vi "Inputs.vi"(8 "error in (no error)":errorcluster, 11 "State in":T1={"State"=enum."Idle", "Start Time"=timestamp(0 s since 1904-01-01), "Configuration"={"Cycle Period"=0.0, "Mettler"={"VISA resource name"="", "Simulated?"=FALSE}, "Scale Type"=""}, "Current Time"=timestamp(0 s since 1904-01-01), "First Iteration"=FALSE, "Data"={"Scale Read(g)"=0.0}, "Process Name"="", "Log Started"=FALSE}) -> (0 "error out":errorcluster, 3 "State out":T1={"State"=enum."Idle", "Start Time"=timestamp(0 s since 1904-01-01), "Configuration"={"Cycle Period"=0.0, "Mettler"={"VISA resource name"="", "Simulated?"=FALSE}, "Scale Type"=""}, "Current Time"=timestamp(0 s since 1904-01-01), "First Iteration"=FALSE, "Data"={"Scale Read(g)"=0.0}, "Process Name"="", "Log Started"=FALSE})   [LabVIEW 2018, in "Sonicator Module.lvlib" / "Sonicator Module Engine.lvlib"]
uses:
  Sonicator Module Engine.lvlib
  State Cluster.ctl
  State Enum.ctl
  Feed Module/Controls/Sonicator Module Settings Cluster.ctl
  Mettler Toledo/Controls/Settings Cluster.ctl
  Tag VIs/Tag FGV Operation Enum.ctl
  Mettler Toledo/Mettler Toledo.lvlib
  Shared Variables/Dynamic Shared Variables.lvlib
  Sonicator Module.lvlib
panel:
  # "Scale Settings"
  # "Scale Settings"
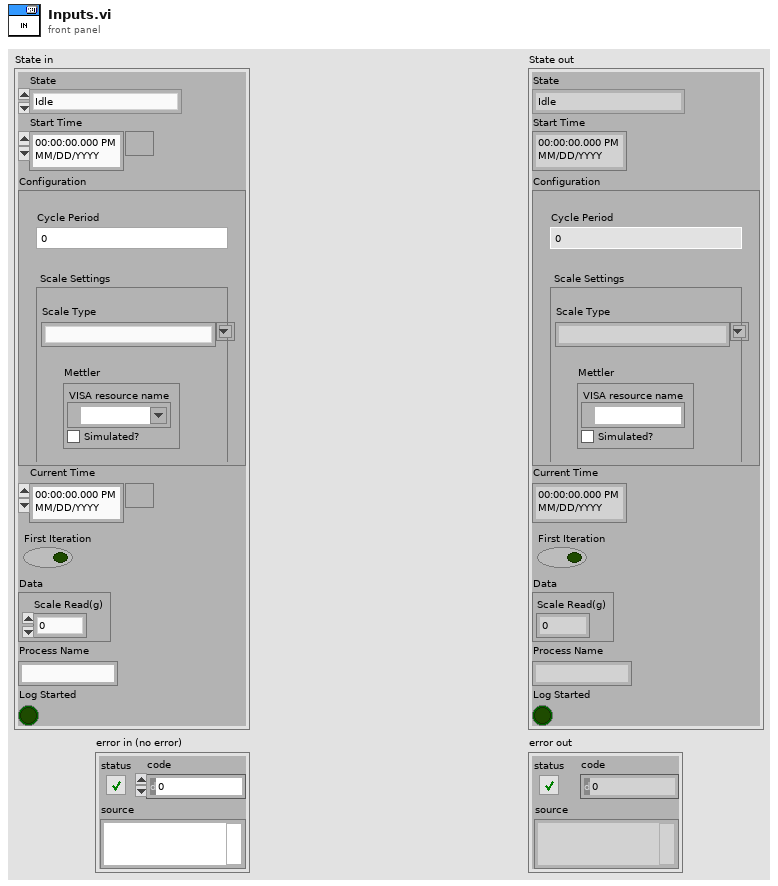
[diagram p1: front panel]
types:
  T1 = typedef "Sonicator Module.lvlib/Sonicator Module Engine.lvlib/State Cluster.ctl" = cluster{"State":T2, "Start Time":timestamp, "Configuration":T3, "Current Time":timestamp, "First Iteration":bool, "Data":cluster{"Scale Read(g)":dbl}, "Process Name":string, "Log Started":bool}
  T2 = typedef "Sonicator Module.lvlib/Sonicator Module Engine.lvlib/State Enum.ctl" = enum16{"Measuring", "Idle"}
  T3 = typedef "Sonicator Module.lvlib/Sonicator Module Settings Cluster.ctl" = cluster{"Cycle Period":dbl, "Mettler":T4, "Scale Type":string}
  T4 = typedef "Mettler Toledo.lvlib/Settings Cluster.ctl" = cluster{"VISA resource name":refnum<visa-resource-name>, "Simulated?":bool}
  T5 = typedef "Tag FGV Operation Enum.ctl" = enum16{"Init", "Set Notification Queue", "Create Tag", "Commit", "Write Tag (Numeric)", "Write Tag (Boolean)", "Read All Tags", "Read One Tag", "Delete Tag Category", "Set Alarm Parameters (Numeric)", "Set Alarm Parameters (Boolean)", "Enable All Alarms", "Disable All Alarms", "Delete All Tags", "Read Alarms", "Ack Alarm", "Read Alarm Parameters (Numeric)", "Read Alarm Parameters (Boolean)"}
  T6 = cluster{"Scale Tag":string, "Output Device Tag":string}
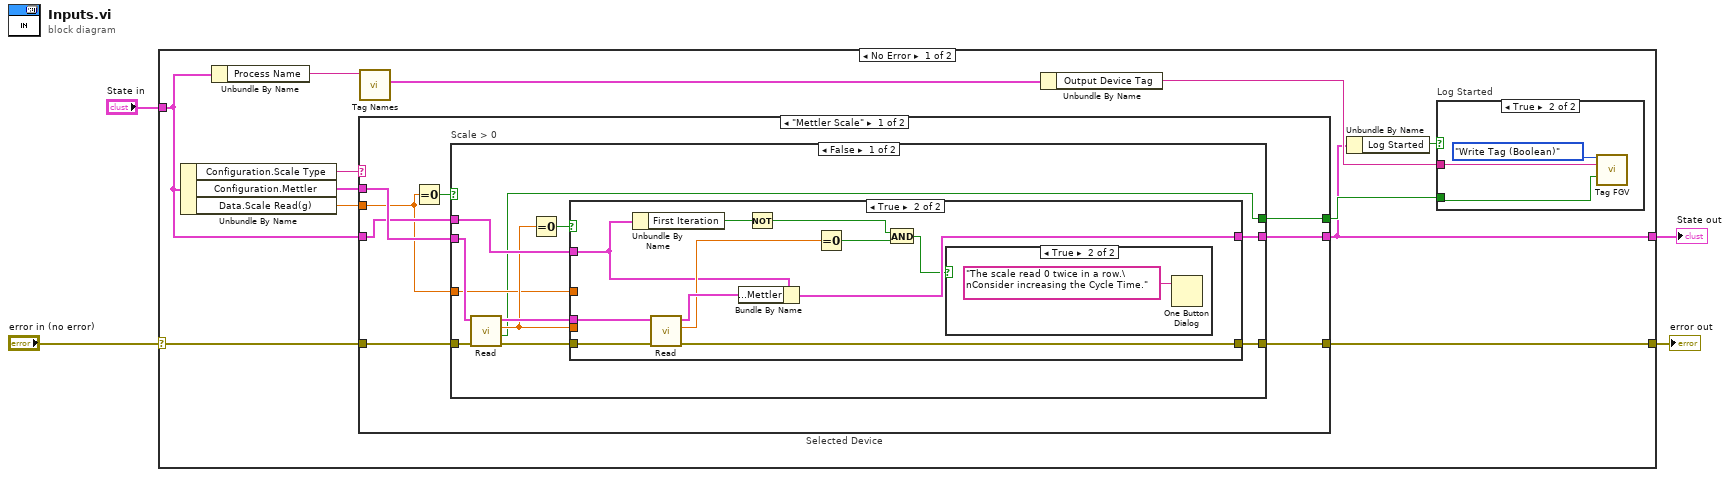
[diagram p0: block diagram]
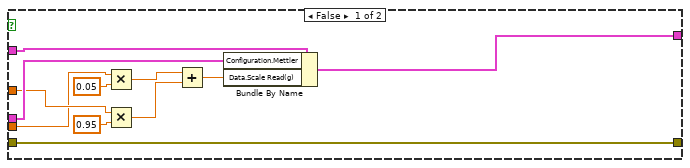
[diagram p3: hidden frame]
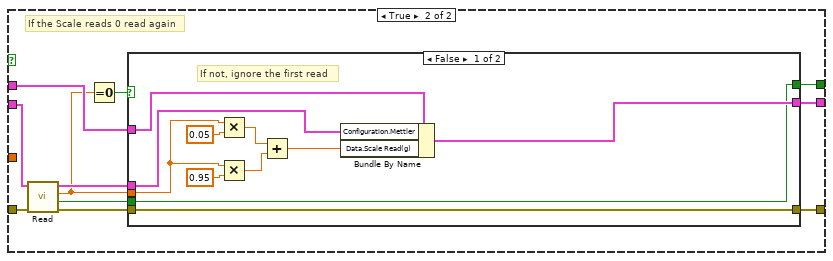
[diagram p5: hidden frame]
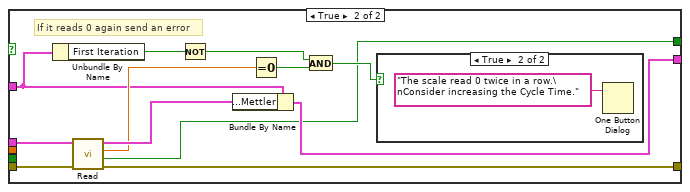
[diagram p6: hidden frame]
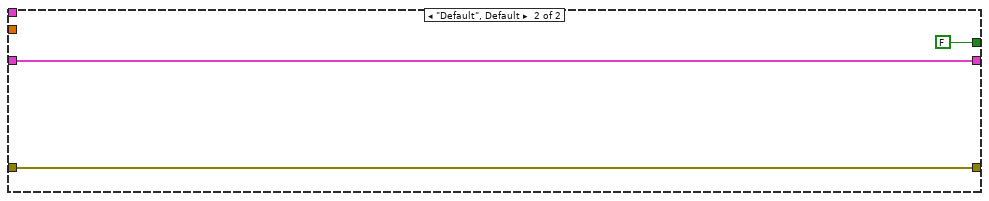
[diagram p8: hidden frame]
diagram:
  n1 = case shown="No Error" "error in (no error)" {
    selector: "error in (no error)" -> [w14 w101]
    tunnel: [w13 w101] -> w1
    tunnel: "State in" -> [w10 w100]
    tunnel: [w6 w100] -> w2
    frame No Error {
      n2 = Unbundle By Name(w10) -> ("Configuration.Scale Type"=w16:string, "Configuration.Mettler"=w15:T4, "Data.Scale Read(g)"=w12:dbl)
      n3 = Unbundle By Name(w10) -> ("Process Name"=w9:string)
      n4 = case "Selected Device" shown="\"Mettler Scale\"" w16 {
        tunnel: w10 -> [w25 w99]
        tunnel: [w24 w99] -> w6
        tunnel: w15 -> [w26 _]
        tunnel: w14 -> [w27 w98]
        tunnel: [w23 w98] -> w13
        tunnel: w12 -> [w22 _]
        tunnel: [w20 FALSE ("Connection Error")] -> w11
        frame "Mettler Scale" {
          n5 = Equal To 0?(x=w22) -> (x = 0?=w21:bool)
          n6 = case "Scale > 0" shown="False" w21 {
            tunnel: w27 -> [w38 w71]
            tunnel: w26 -> [w37 w72]
            tunnel: w25 -> [w34 w68]
            tunnel: [w32 w65] -> w24
            tunnel: [w30 w64] -> w23
            tunnel: w22 -> [w29 _]
            tunnel: [w28 w63] -> w20
            frame False {
              n7 = call "Read.vi"("error in (no error)"=w38, "Mettler Settings in"=w37) -> ("error out"=w31:errorcluster, "Connection Error"=w28:bool, "mass (g)"=w33:dbl, "Mettler Settings out"=w35:T4)  [unwired: 6 in]
              n8 = Equal To 0?(x=w33) -> (x = 0?=w36:bool)
              n9 = case shown="True" w36 {
                tunnel: w33 -> [w39 _]
                tunnel: w34 -> [w49 w55]
                tunnel: w35 -> [w48 w59]
                tunnel: [w47 w60] -> w32
                tunnel: w31 -> [w46 w57]
                tunnel: [w46 w50] -> w30
                tunnel: w29 -> [w40 _]
                frame False {
                  n10 = Multiply(x=w39, y=0.05) -> (x*y=w42:dbl)
                  n11 = Multiply(x=w40, y=0.95) -> (x*y=w45:dbl)
                  n12 = Add(x=w42, y=w45) -> (x+y=w41:dbl)
                  n13 = Bundle By Name(cluster=w49, "Configuration.Mettler"=w48, "Data.Scale Read(g)"=w41) -> (w47:T1)
                }
                frame True {
                  n14 = Unbundle By Name(w55) -> ("First Iteration"=w54:bool)
                  n15 = call "Read.vi"("error in (no error)"=w57, "Mettler Settings in"=w59) -> ("error out"=w50:errorcluster, "mass (g)"=w56:dbl, "Mettler Settings out"=w58:T4)  [unwired: 6 in, 1 out]
                  n16 = Bundle By Name(cluster=w55, "Configuration.Mettler"=w58) -> (w60:T1)
                  n17 = Not(x=w54) -> (.not. x?=w53:bool)
                  n18 = Equal To 0?(x=w56) -> (x = 0?=w52:bool)
                  n19 = And(x=w53, y=w52) -> (x .and. y?=w51:bool)
                  n20 = case shown="True" w51 {
                    frame False {
                    }
                    frame True {
                      n21 = One Button Dialog(message="The scale read 0 twice in a row.\nConsider increasing the Cycle Time.") -> ()  [unwired: 1 in, 1 out]
                    }
                  }
                }
              }
            }
            frame True {
              # "If the Scale reads 0 read again"
              n22 = call "Read.vi"("error in (no error)"=w71, "Mettler Settings in"=w72) -> ("error out"=w67:errorcluster, "Connection Error"=w62:bool, "mass (g)"=w66:dbl, "Mettler Settings out"=w69:T4)  [unwired: 6 in]
              n23 = Equal To 0?(x=w66) -> (x = 0?=w70:bool)
              n24 = case shown="False" w70 {
                tunnel: w66 -> [w74 _]
                tunnel: w68 -> [w83 w90]
                tunnel: w69 -> [w82 w94]
                tunnel: [w81 w95] -> w65
                tunnel: w67 -> [w80 w92]
                tunnel: [w80 w85] -> w64
                tunnel: [w73 w84] -> w63
                tunnel: w62 -> [w73 _]
                frame False {
                  # "If not, ignore the first read"
                  n25 = Multiply(x=w74, y=0.05) -> (x*y=w76:dbl)
                  n26 = Multiply(x=w74, y=0.95) -> (x*y=w79:dbl)
                  n27 = Add(x=w76, y=w79) -> (x+y=w75:dbl)
                  n28 = Bundle By Name(cluster=w83, "Configuration.Mettler"=w82, "Data.Scale Read(g)"=w75) -> (w81:T1)
                }
                frame True {
                  # "If it reads 0 again send an error"
                  n29 = Unbundle By Name(w90) -> ("First Iteration"=w89:bool)
                  n30 = call "Read.vi"("error in (no error)"=w92, "Mettler Settings in"=w94) -> ("error out"=w85:errorcluster, "Connection Error"=w84:bool, "mass (g)"=w91:dbl, "Mettler Settings out"=w93:T4)  [unwired: 6 in]
                  n31 = Not(x=w89) -> (.not. x?=w88:bool)
                  n32 = Bundle By Name(cluster=w90, "Configuration.Mettler"=w93) -> (w95:T1)
                  n33 = Equal To 0?(x=w91) -> (x = 0?=w87:bool)
                  n34 = And(x=w88, y=w87) -> (x .and. y?=w86:bool)
                  n35 = case shown="True" w86 {
                    frame False {
                    }
                    frame True {
                      n36 = One Button Dialog(message="The scale read 0 twice in a row.\nConsider increasing the Cycle Time.") -> ()  [unwired: 1 in, 1 out]
                    }
                  }
                }
              }
            }
          }
        }
        frame "Default", Default {
        }
      }
      n37 = call "Tag Names.vi"("Process Name"=w9) -> ("Scale Tags"=w8:T6)  [unwired: 8 in, 2 out]
      n38 = Unbundle By Name(w8) -> ("Output Device Tag"=w7:string)
      n39 = Unbundle By Name(w6) -> ("Log Started"=w5:bool)
      n40 = case "Log Started" shown="True" w5 {
        tunnel: w11 -> [_ w17]
        tunnel: w7 -> [_ w18]
        frame False {
        }
        frame True {
          n41 = call "Tag FGV.vi"("Operation"=Tag_FGV_Operation_Enum."Write Tag (Boolean)", "Tag Name"=w18, "Data"=w17) -> ()  [unwired: 5 in, 8 out]
        }
      }
    }
    frame Error {
    }
  }
  "error out" <- w1
  "State out" <- w2
